vi "Weather Parse Test.vi"() -> ()   [LabVIEW 2020, in "CDM-Config.lvlib"] (continued)
                      \"CMAS\"\n                    ],\n                    \"VTEC\": [\n                        \"/O.CON.KDLH.SC.Y.0132.000000T0000Z-251204T1800Z/\"\n                    ],\n                    \"eventEndingTime\": [\n                        \"2025-12-04T12:00:00-06:00\"\n                    ],\n                    \"expiredReferences\": [\n                        \"w-nws.webmaster@noaa.gov,urn:oid:2.49.0.1.840.0.04f9cf691f6928c5262dfbb988fe18619f2f30e0.003.1,2025-12-02T21:23:00-06:00 w-nws.webmaster@noaa.gov,urn:oid:2.49.0.1.840.0.d19370faedd72659268a7c7b3bafbf3617bad502.003.1,2025-12-02T15:02:00-06:00 w-nws.webmaster@noaa.gov,urn:oid:2.49.0.1.840.0.21fbf4d0662dfb62d7facea472c0c3fe427de6a4.001.1,2025-12-02T09:49:00-06:00\"\n                    ]\n                },\n                \"scope\": \"Public\",\n                \"code\": \"IPAWSv1.0\",\n                \"language\": \"en-US\",\n                \"web\": \"http://www.weather.gov\",\n                \"eventCode\": {\n                    \"SAME\": [\n                        \"NWS\"\n                    ],\n                    \"NationalWeatherService\": [\n                        \"SCY\"\n                    ]\n                }\n            }\n        },\n        {\n            \"id\": \"https://api.weather.gov/alerts/urn:oid:2.49.0.1.840.0.4a9c30a731508078f0f7520ff08e9f1f7a671578.003.2\",\n            \"type\": \"Feature\",\n            \"geometry\": null,\n            \"properties\": {\n                \"@id\": \"https://api.weather.gov/alerts/urn:oid:2.49.0.1.840.0.4a9c30a731508078f0f7520ff08e9f1f7a671578.003.2\",\n                \"@type\": \"wx:Alert\",\n                \"id\": \"urn:oid:2.49.0.1.840.0.4a9c30a731508078f0f7520ff08e9f1f7a671578.003.2\",\n                \"areaDesc\": \"Silver Bay Harbor to Two Harbors MN; Two Harbors to Duluth MN\",\n                \"geocode\": {\n                    \"SAME\": [\n                        \"091143\",\n                        \"091144\"\n                    ],\n                    \"UGC\": [\n                        \"LSZ143\",\n                        \"LSZ144\"\n                    ]\n                },\n                \"affectedZones\": [\n                    \"https://api.weather.gov/zones/forecast/LSZ143\",\n                    \"https://api.weather.gov/zones/forecast/LSZ144\"\n                ],\n                \"references\": [\n                    {\n                        \"@id\": \"https://api.weather.gov/alerts/urn:oid:2.49.0.1.840.0.2b3611bf51a8d91812a27a6d34dc1646d3578776.003.2\",\n                        \"identifier\": \"urn:oid:2.49.0.1.840.0.2b3611bf51a8d91812a27a6d34dc1646d3578776.003.2\",\n                        \"sender\": \"w-nws.webmaster@noaa.gov\",\n                        \"sent\": \"2025-12-03T04:05:00-06:00\"\n                    }\n                ],\n                \"sent\": \"2025-12-03T09:55:00-06:00\",\n                \"effective\": \"2025-12-03T09:55:00-06:00\",\n                \"onset\": \"2025-12-04T12:00:00-06:00\",\n                \"expires\": \"2025-12-03T22:00:00-06:00\",\n                \"ends\": \"2025-12-05T00:00:00-06:00\",\n                \"status\": \"Actual\",\n                \"messageType\": \"Update\",\n                \"category\": \"Met\",\n                \"severity\": \"Moderate\",\n                \"certainty\": \"Possible\",\n                \"urgency\": \"Future\",\n                \"event\": \"Gale Watch\",\n                \"sender\": \"w-nws.webmaster@noaa.gov\",\n                \"senderName\": \"NWS Duluth MN\",\n                \"headline\": \"Gale Watch issued December 3 at 9:55AM CST until December 5 at 12:00AM CST by NWS Duluth MN\",\n                \"description\": \"* WHAT...For the Small Craft Advisory, west winds 10 to 20 kt\\nwith gusts up to 25 kt and waves 1 to 2 ft. For the Gale\\nWatch, southwest winds 15 to 25 kt with gusts up to 35 kt and\\nwaves 3 to 6 ft possible.\\n\\n* WHERE...Silver Bay Harbor to Two Harbors MN and Two Harbors to\\nDuluth MN.\\n\\n* WHEN...For the Small Craft Advisory, until noon CST Thursday.\\nFor the Gale Watch, from Thursday afternoon through Thursday\\nevening.\\n\\n* IMPACTS...Strong winds can cause hazardous waves which could\\ncapsize or damage vessels and reduce visibility.\\n\\n* ADDITIONAL DETAILS...Wind gusts may drop below 20 knots for a\\ntime early this morning and again Thursday morning.\",\n                \"instruction\": \"Mariners should consider altering plans to avoid possible\\nhazardous conditions.  Remain in port, seek safe harbor, alter\\ncourse, and/or secure the vessel for severe wind and waves.\",\n                \"response\": \"Prepare\",\n                \"parameters\": {\n                    \"AWIPSidentifier\": [\n                        \"MWWDLH\"\n                    ],\n                    \"WMOidentifier\": [\n                        \"WHUS73 KDLH 031555\"\n                    ],\n                    \"NWSheadline\": [\n                        \"SMALL CRAFT ADVISORY REMAINS IN EFFECT UNTIL NOON CST THURSDAY... ...GALE WATCH REMAINS IN EFFECT FROM THURSDAY AFTERNOON THROUGH THURSDAY EVENING\"\n                    ],\n                    \"BLOCKCHANNEL\": [\n                        \"EAS\",\n                        \"NWEM\",\n                        \"CMAS\"\n                    ],\n                    \"VTEC\": [\n                        \"/O.CON.KDLH.GL.A.0018.251204T1800Z-251205T0600Z/\"\n                    ],\n                    \"eventEndingTime\": [\n                        \"2025-12-05T00:00:00-06:00\"\n                    ],\n                    \"expiredReferences\": [\n                        \"w-nws.webmaster@noaa.gov,urn:oid:2.49.0.1.840.0.04f9cf691f6928c5262dfbb988fe18619f2f30e0.003.2,2025-12-02T21:23:00-06:00\"\n                    ]\n                },\n                \"scope\": \"Public\",\n                \"code\": \"IPAWSv1.0\",\n                \"language\": \"en-US\",\n                \"web\": \"http://www.weather.gov\",\n                \"eventCode\": {\n                    \"SAME\": [\n                        \"NWS\"\n                    ],\n                    \"NationalWeatherService\": [\n                        \"GLA\"\n                    ]\n                }\n            }\n        },\n        {\n            \"id\": \"https://api.weather.gov/alerts/urn:oid:2.49.0.1.840.0.4a9c30a731508078f0f7520ff08e9f1f7a671578.002.2\",\n            \"type\": \"Feature\",\n            \"geometry\": null,\n            \"properties\": {\n                \"@id\": \"https://api.weather.gov/alerts/urn:oid:2.49.0.1.840.0.4a9c30a731508078f0f7520ff08e9f1f7a671578.002.2\",\n                \"@type\": \"wx:Alert\",\n                \"id\": \"urn:oid:2.49.0.1.840.0.4a9c30a731508078f0f7520ff08e9f1f7a671578.002.2\",\n                \"areaDesc\": \"Grand Portage to Grand Marais MN; Grand Marais to Taconite Harbor MN; Taconite Harbor to Silver Bay Harbor MN\",\n                \"geocode\": {\n                    \"SAME\": [\n                        \"091140\",\n                        \"091141\",\n                        \"091142\"\n                    ],\n                    \"UGC\": [\n                        \"LSZ140\",\n                        \"LSZ141\",\n                        \"LSZ142\"\n                    ]\n                },\n                \"affectedZones\": [\n                    \"https://api.weather.gov/zones/forecast/LSZ140\",\n                    \"https://api.weather.gov/zones/forecast/LSZ141\",\n                    \"https://api.weather.gov/zones/forecast/LSZ142\"\n                ],\n                \"references\": [\n                    {\n                        \"@id\": \"https://api.weather.gov/alerts/urn:oid:2.49.0.1.840.0.2b3611bf51a8d91812a27a6d34dc1646d3578776.002.2\",\n                        \"identifier\": \"urn:oid:2.49.0.1.840.0.2b3611bf51a8d91812a27a6d34dc1646d3578776.002.2\",\n                        \"sender\": \"w-nws.webmaster@noaa.gov\",\n                        \"sent\": \"2025-12-03T04:05:00-06:00\"\n                    }\n                ],\n                \"sent\": \"2025-12-03T09:55:00-06:00\",\n                \"effective\": \"2025-12-03T09:55:00-06:00\",\n                \"onset\": \"2025-12-04T12:00:00-06:00\",\n                \"expires\": \"2025-12-03T22:00:00-06:00\",\n                \"ends\": \"2025-12-05T00:00:00-06:00\",\n                \"status\": \"Actual\",\n                \"messageType\": \"Update\",\n                \"category\": \"Met\",\n                \"severity\": \"Moderate\",\n                \"certainty\": \"Possible\",\n                \"urgency\": \"Future\",\n                \"event\": \"Gale Watch\",\n                \"sender\": \"w-nws.webmaster@noaa.gov\",\n                \"senderName\": \"NWS Duluth MN\",\n                \"headline\": \"Gale Watch issued December 3 at 9:55AM CST until December 5 at 12:00AM CST by NWS Duluth MN\",\n                \"description\": \"* WHAT...For the Small Craft Advisory, northwest winds 10 to 20\\nkt with gusts up to 30 kt and waves 1 to 2 ft. For the Gale\\nWatch, southwest winds 15 to 25 kt with gusts up to 35 kt and\\nwaves 6 to 9 ft possible.\\n\\n* WHERE...Grand Portage to Grand Marais MN, Grand Marais to\\nTaconite Harbor MN and Taconite Harbor to Silver Bay Harbor MN.\\n\\n* WHEN...For the Small Craft Advisory, until noon CST Thursday.\\nFor the Gale Watch, from Thursday afternoon through Thursday\\nevening.\\n\\n* IMPACTS...Strong winds can cause hazardous waves which could\\ncapsize or damage vessels and reduce visibility.\\n\\n* ADDITIONAL DETAILS...Wind gusts may drop below 20 knots for a\\ntime early this morning and again Thursday morning.\",\n                \"instruction\": \"Mariners should consider altering plans to avoid possible\\nhazardous conditions.  Remain in port, seek safe harbor, alter\\ncourse, and/or secure the vessel for severe wind and waves.\",\n                \"response\": \"Prepare\",\n                \"parameters\": {\n                    \"AWIPSidentifier\": [\n                        \"MWWDLH\"\n                    ],\n                    \"WMOidentifier\": [\n                        \"WHUS73 KDLH 031555\"\n                    ],\n                    \"NWSheadline\": [\n                        \"SMALL CRAFT ADVISORY REMAINS IN EFFECT UNTIL NOON CST THURSDAY... ...GALE WATCH REMAINS IN EFFECT FROM THURSDAY AFTERNOON THROUGH THURSDAY EVENING\"\n                    ],\n                    \"BLOCKCHANNEL\": [\n                        \"EAS\",\n                        \"NWEM\",\n                        \"CMAS\"\n                    ],\n                    \"VTEC\": [\n                        \"/O.CON.KDLH.GL.A.0018.251204T1800Z-251205T0600Z/\"\n                    ],\n                    \"eventEndingTime\": [\n                        \"2025-12-05T00:00:00-06:00\"\n                    ],\n                    \"expiredReferences\": [\n                        \"w-nws.webmaster@noaa.gov,urn:oid:2.49.0.1.840.0.04f9cf691f6928c5262dfbb988fe18619f2f30e0.002.2,2025-12-02T21:23:00-06:00\"\n                    ]\n                },\n                \"scope\": \"Public\",\n                \"code\": \"IPAWSv1.0\",\n                \"language\": \"en-US\",\n                \"web\": \"http://www.weather.gov\",\n                \"eventCode\": {\n                    \"SAME\": [\n                        \"NWS\"\n                    ],\n                    \"NationalWeatherService\": [\n                        \"GLA\"\n                    ]\n                }\n            }\n        },\n        {\n            \"id\": \"https://api.weather.gov/alerts/urn:oid:2.49.0.1.840.0.4a9c30a731508078f0f7520ff08e9f1f7a671578.004.1\",\n            \"type\": \"Feature\",\n            \"geometry\": null,\n            \"properties\": {\n                \"@id\": \"https://api.weather.gov/alerts/urn:oid:2.49.0.1.840.0.4a9c30a731508078f0f7520ff08e9f1f7a671578.004.1\",\n                \"@type\": \"wx:Alert\",\n                \"id\": \"urn:oid:2.49.0.1.840.0.4a9c30a731508078f0f7520ff08e9f1f7a671578.004.1\",\n                \"areaDesc\": \"Chequamegon Bay-Bayfield to Oak Point WI; Duluth MN to Port Wing WI; Port Wing to Sand Island WI; Sand Island to Bayfield WI; Oak Point to Saxon Harbor WI\",\n                \"geocode\": {\n                    \"SAME\": [\n                        \"091121\",\n                        \"091145\",\n                        \"091146\",\n                        \"091147\",\n                        \"091148\"\n                    ],\n                    \"UGC\": [\n                        \"LSZ121\",\n                        \"LSZ145\",\n                        \"LSZ146\",\n                        \"LSZ147\",\n                        \"LSZ148\"\n                    ]\n                },\n                \"affectedZones\": [\n                    \"https://api.weather.gov/zones/forecast/LSZ121\",\n                    \"https://api.weather.gov/zones/forecast/LSZ145\",\n                    \"https://api.weather.gov/zones/forecast/LSZ146\",\n                    \"https://api.weather.gov/zones/forecast/LSZ147\",\n                    \"https://api.weather.gov/zones/forecast/LSZ148\"\n                ],\n                \"references\": [\n                    {\n                        \"@id\": \"https://api.weather.gov/alerts/urn:oid:2.49.0.1.840.0.2b3611bf51a8d91812a27a6d34dc1646d3578776.004.1\",\n                        \"identifier\": \"urn:oid:2.49.0.1.840.0.2b3611bf51a8d91812a27a6d34dc1646d3578776.004.1\",\n                        \"sender\": \"w-nws.webmaster@noaa.gov\",\n                        \"sent\": \"2025-12-03T04:05:00-06:00\"\n                    }\n                ],\n                \"sent\": \"2025-12-03T09:55:00-06:00\",\n                \"effective\": \"2025-12-03T09:55:00-06:00\",\n                \"onset\": \"2025-12-03T09:55:00-06:00\",\n                \"expires\": \"2025-12-03T22:00:00-06:00\",\n                \"ends\": \"2025-12-05T10:00:00-06:00\",\n                \"status\": \"Actual\",\n                \"messageType\": \"Update\",\n                \"category\": \"Met\",\n                \"severity\": \"Minor\",\n                \"certainty\": \"Likely\",\n                \"urgency\": \"Expected\",\n                \"event\": \"Small Craft Advisory\",\n                \"sender\": \"w-nws.webmaster@noaa.gov\",\n                \"senderName\": \"NWS Duluth MN\",\n                \"headline\": \"Small Craft Advisory issued December 3 at 9:55AM CST until December 5 at 10:00AM CST by NWS Duluth MN\",\n                \"description\": \"* WHAT...West winds 15 to 25 kt with gusts up to 35 kt and waves\\n2 to 5 ft.\\n\\n* WHERE...Chequamegon Bay-Bayfield to Oak Point WI, Duluth MN to\\nPort Wing WI, Port Wing to Sand Island WI, Sand Island to\\nBayfield WI and Oak Point to Saxon Harbor WI.\\n\\n* WHEN...Until 10 AM CST Friday.\\n\\n* IMPACTS...Conditions will be hazardous to small craft.\\n\\n* ADDITIONAL DETAILS...Wind gusts may drop below 20 knots for a\\ntime early this morning and again Thursday morning.\",\n                \"instruction\": \"Anyone operating a smaller vessel should avoid navigating in\\nhazardous conditions.\",\n                \"response\": \"Avoid\",\n                \"parameters\": {\n                    \"AWIPSidentifier\": [\n                        \"MWWDLH\"\n                    ],\n                    \"WMOidentifier\": [\n                        \"WHUS73 KDLH 031555\"\n                    ],\n                    \"NWSheadline\": [\n                        \"SMALL CRAFT ADVISORY REMAINS IN EFFECT UNTIL 10 AM CST FRIDAY\"\n                    ],\n                    \"BLOCKCHANNEL\": [\n                        \"EAS\",\n                        \"NWEM\",\n                        \"CMAS\"\n                    ],\n                    \"VTEC\": [\n                        \"/O.CON.KDLH.SC.Y.0132.000000T0000Z-251205T1600Z/\"\n                    ],\n                    \"eventEndingTime\": [\n                        \"2025-12-05T10:00:00-06:00\"\n                    ],\n                    \"expiredReferences\": [\n                        \"w-nws.webmaster@noaa.gov,urn:oid:2.49.0.1.840.0.04f9cf691f6928c5262dfbb988fe18619f2f30e0.004.1,2025-12-02T21:23:00-06:00 w-nws.webmaster@noaa.gov,urn:oid:2.49.0.1.840.0.d19370faedd72659268a7c7b3bafbf3617bad502.003.1,2025-12-02T15:02:00-06:00 w-nws.webmaster@noaa.gov,urn:oid:2.49.0.1.840.0.21fbf4d0662dfb62d7facea472c0c3fe427de6a4.001.1,2025-12-02T09:49:00-06:00\"\n                    ]\n                },\n                \"scope\": \"Public\",\n                \"code\": \"IPAWSv1.0\",\n                \"language\": \"en-US\",\n                \"web\": \"http://www.weather.gov\",\n                \"eventCode\": {\n                    \"SAME\": [\n                        \"NWS\"\n                    ],\n                    \"NationalWeatherService\": [\n                        \"SCY\"\n                    ]\n                }\n            }\n        },\n        {\n            \"id\": \"https://api.weather.gov/alerts/urn:oid:2.49.0.1.840.0.cb3741455a35586feac70bfcfc92a33545eb4f89.001.1\",\n            \"type\": \"Feature\",\n            \"geometry\": null,\n            \"properties\": {\n                \"@id\": \"https://api.weather.gov/alerts/urn:oid:2.49.0.1.840.0.cb3741455a35586feac70bfcfc92a33545eb4f89.001.1\",\n                \"@type\": \"wx:Alert\",\n                \"id\": \"urn:oid:2.49.0.1.840.0.cb3741455a35586feac70bfcfc92a33545eb4f89.001.1\",\n                \"areaDesc\": \"Southern Blue Mountains of Oregon; John Day Basin; Ochoco-John Day Highlands; North Central Oregon\",\n                \"geocode\": {\n                    \"SAME\": [\n                        \"041021\",\n                        \"041023\",\n                        \"041049\",\n                        \"041059\",\n                        \"041061\",\n                        \"041069\",\n                        \"041031\",\n                        \"041065\",\n                        \"041013\",\n                        \"041017\",\n                        \"041055\"\n                    ],\n                    \"UGC\": [\n                        \"ORZ503\",\n                        \"ORZ505\",\n                        \"ORZ506\",\n                        \"ORZ510\"\n                    ]\n                },\n                \"affectedZones\": [\n                    \"https://api.weather.gov/zones/forecast/ORZ503\",\n                    \"https://api.weather.gov/zones/forecast/ORZ505\",\n                    \"https://api.weather.gov/zones/forecast/ORZ506\",\n                    \"https://api.weather.gov/zones/forecast/ORZ510\"\n                ],\n                \"references\": [],\n                \"sent\": \"2025-12-03T07:47:00-08:00\",\n                \"effective\": \"2025-12-03T07:47:00-08:00\",\n                \"onset\": \"2025-12-03T07:47:00-08:00\",\n                \"expires\": \"2025-12-03T13:00:00-08:00\",\n                \"ends\": null,\n                \"status\": \"Actual\",\n                \"messageType\": \"Alert\",\n                \"category\": \"Met\",\n                \"severity\": \"Moderate\",\n                \"certainty\": \"Observed\",\n                \"urgency\": \"Expected\",\n                \"event\": \"Special Weather Statement\",\n                \"sender\": \"w-nws.webmaster@noaa.gov\",\n                \"senderName\": \"NWS Pendleton OR\",\n                \"headline\": \"Special Weather Statement issued December 3 at 7:47AM PST by NWS Pendleton OR\",\n                \"description\": \"Patchy dense freezing fog has been observed on local traffic and\\nwildfire cameras, with visibilities estimated to be less than a\\nmile and temperatures below freezing in some of these areas. Area\\nhighways that are being impacted include US Highways 395, 97,\\n197, 26, and 20, as well as Oregon Highways 218, 216, 208, 207,\\n206, 74, and 19. Reduced visibilities and ice accretion on\\nroadways may impact travel. The freezing fog will lift by this\\nafternoon.\",\n                \"instruction\": null,\n                \"response\": \"Execute\",\n                \"parameters\": {\n                    \"AWIPSidentifier\": [\n                        \"SPSPDT\"\n                    ],\n                    \"WMOidentifier\": [\n                        \"WWUS86 KPDT 031547\"\n                    ],\n                    \"BLOCKCHANNEL\": [\n                        \"EAS\",\n                        \"NWEM\",\n                        \"CMAS\"\n                    ],\n                    \"EAS-ORG\": [\n                        \"WXR\"\n                    ]\n                },\n                \"scope\": \"Public\",\n                \"code\": \"IPAWSv1.0\",\n                \"language\": \"en-US\",\n                \"web\": \"http://www.weather.gov\",\n                \"eventCode\": {\n                    \"SAME\": [\n                        \"SPS\"\n                    ],\n                    \"NationalWeatherService\": [\n                        \"SPS\"\n                    ]\n                }\n            }\n        },\n        {\n            \"id\": \"https://api.weather.gov/alerts/urn:oid:2.49.0.1.840.0.d69e0fdad84e1f558091761919060d14ba7d6a4a.001.1\",\n            \"type\": \"Feature\",\n            \"geometry\": null,\n            \"properties\": {\n                \"@id\": \"https://api.weather.gov/alerts/urn:oid:2.49.0.1.840.0.d69e0fdad84e1f558091761919060d14ba7d6a4a.001.1\",\n                \"@type\": \"wx:Alert\",\n                \"id\": \"urn:oid:2.49.0.1.840.0.d69e0fdad84e1f558091761919060d14ba7d6a4a.001.1\",\n                \"areaDesc\": \"Grand Traverse Bay south of a line Grand Traverse Light to Norwood MI; Seul Choix Point to 5NM West of Mackinac Bridge; Norwood MI to 5NM West of Mackinac Bridge including Little Traverse Bay; Sleeping Bear Point to Grand Traverse Light MI; Point Betsie to Sleeping Bear Point MI; Manistee to Point Betsie MI\",\n                \"geocode\": {\n                    \"SAME\": [\n                        \"092323\",\n                        \"092341\",\n                        \"092342\",\n                        \"092344\",\n                        \"092345\",\n                        \"092346\"\n                    ],\n                    \"UGC\": [\n                        \"LMZ323\",\n                        \"LMZ341\",\n                        \"LMZ342\",\n                        \"LMZ344\",\n                        \"LMZ345\",\n                        \"LMZ346\"\n                    ]\n                },\n                \"affectedZones\": [\n                    \"https://api.weather.gov/zones/forecast/LMZ323\",\n                    \"https://api.weather.gov/zones/forecast/LMZ341\",\n                    \"https://api.weather.gov/zones/forecast/LMZ342\",\n                    \"https://api.weather.gov/zones/forecast/LMZ344\",\n                    \"https://api.weather.gov/zones/forecast/LMZ345\",\n                    \"https://api.weather.gov/zones/forecast/LMZ346\"\n                ],\n                \"references\": [\n                    {\n                        \"@id\": \"https://api.weather.gov/alerts/urn:oid:2.49.0.1.840.0.d4f341bf09774259e03e3637f08a5e0369a8be29.001.1\",\n                        \"identifier\": \"urn:oid:2.49.0.1.840.0.d4f341bf09774259e03e3637f08a5e0369a8be29.001.1\",\n                        \"sender\": \"w-nws.webmaster@noaa.gov\",\n                        \"sent\": \"2025-12-03T02:58:00-05:00\"\n                    }\n                ],\n                \"sent\": \"2025-12-03T10:45:00-05:00\",\n                \"effective\": \"2025-12-03T10:45:00-05:00\",\n                \"onset\": \"2025-12-03T10:45:00-05:00\",\n                \"expires\": \"2025-12-03T19:45:00-05:00\",\n                \"ends\": \"2025-12-04T13:00:00-05:00\",\n                \"status\": \"Actual\",\n                \"messageType\": \"Update\",\n                \"category\": \"Met\",\n                \"severity\": \"Minor\",\n                \"certainty\": \"Likely\",\n                \"urgency\": \"Expected\",\n                \"event\": \"Small Craft Advisory\",\n                \"sender\": \"w-nws.webmaster@noaa.gov\",\n                \"senderName\": \"NWS Gaylord MI\",\n                \"headline\": \"Small Craft Advisory issued December 3 at 10:45AM EST until December 4 at 1:00PM EST by NWS Gaylord MI\",\n                \"description\": \"* WHAT...For the Small Craft Advisory, Highest gusts up to 30\\nkts from the northwest and highest waves around 8 feet. For\\nthe Gale Watch, Highest gusts up to 45 kts from the southwest\\nand highest waves around 13 feet possible.\\n\\n* WHERE...Portions of Lake Michigan.\\n\\n* WHEN...For the Small Craft Advisory, until 1 PM EST Thursday.\\nFor the Gale Watch, from Thursday evening through Friday\\nmorning.\\n\\n* IMPACTS...Strong winds can cause hazardous highest waves which\\ncould capsize or damage vessels and reduce visibility.\",\n                \"instruction\": \"Mariners should consider altering plans to avoid possible\\nhazardous conditions.  Remain in port, seek safe harbor, alter\\ncourse, and/or secure the vessel for severe wind and highest\\nwaves.\",\n                \"response\": \"Avoid\",\n                \"parameters\": {\n                    \"AWIPSidentifier\": [\n                        \"MWWAPX\"\n                    ],\n                    \"WMOidentifier\": [\n                        \"WHUS73 KAPX 031545\"\n                    ],\n                    \"NWSheadline\": [\n                        \"SMALL CRAFT ADVISORY REMAINS IN EFFECT UNTIL 1 PM EST THURSDAY... ...GALE WATCH REMAINS IN EFFECT FROM THURSDAY EVENING THROUGH FRIDAY MORNING\"\n                    ],\n                    \"BLOCKCHANNEL\": [\n                        \"EAS\",\n                        \"NWEM\",\n                        \"CMAS\"\n                    ],\n                    \"VTEC\": [\n                        \"/O.CON.KAPX.SC.Y.0118.000000T0000Z-251204T1800Z/\"\n                    ],\n                    \"eventEndingTime\": [\n                        \"2025-12-04T13:00:00-05:00\"\n                    ],\n                    \"expiredReferences\": [\n                        \"w-nws.webmaster@noaa.gov,urn:oid:2.49.0.1.840.0.db358447f299fb9ab627f5ec5bd8edba51730923.002.1,2025-12-02T23:15:00-05:00 w-nws.webmaster@noaa.gov,urn:oid:2.49.0.1.840.0.dbbd5f9aa1adb1588c67ea3394dc6c72c6a93051.001.1,2025-12-02T14:38:00-05:00 w-nws.webmaster@noaa.gov,urn:oid:2.49.0.1.840.0.bcebcfef404dc927a35a81355eb23e28922a6e4b.001.1,2025-12-02T10:30:00-05:00 w-nws.webmaster@noaa.gov,urn:oid:2.49.0.1.840.0.0625dac845521af5ccf69b7232976b528a83340a.001.1,2025-12-02T02:46:00-05:00\"\n                    ]\n                },\n                \"scope\": \"Public\",\n                \"code\": \"IPAWSv1.0\",\n                \"language\": \"en-US\",\n                \"web\": \"http://www.weather.gov\",\n                \"eventCode\": {\n                    \"SAME\": [\n                        \"NWS\"\n                    ],\n                    \"NationalWeatherService\": [\n                        \"SCY\"\n                    ]\n                }\n            }\n        },\n        {\n            \"id\": \"https://api.weather.gov/alerts/urn:oid:2.49.0.1.840.0.d69e0fdad84e1f558091761919060d14ba7d6a4a.003.1\",\n            \"type\": \"Feature\",\n            \"geometry\": null,\n            \"properties\": {\n                \"@id\": \"https://api.weather.gov/alerts/urn:oid:2.49.0.1.840.0.d69e0fdad84e1f558091761919060d14ba7d6a4a.003.1\",\n                \"@type\": \"wx:Alert\",\n                \"id\": \"urn:oid:2.49.0.1.840.0.d69e0fdad84e1f558091761919060d14ba7d6a4a.003.1\",\n                \"areaDesc\": \"Straits of Mackinac within 5 nm of Mackinac Bridge including Mackinac Island; St Ignace to False Detour Channel; 5NM East of Mackinac Bridge to Presque Isle Light MI including Bois Blanc Island; Presque Isle Light to Sturgeon Pt MI Including Thunder Bay National Marine Sanctuary; Sturgeon Pt to Alabaster MI\",\n                \"geocode\": {\n                    \"SAME\": [\n                        \"093345\",\n                        \"093346\",\n                        \"093347\",\n                        \"093348\",\n                        \"093349\"\n                    ],\n                    \"UGC\": [\n                        \"LHZ345\",\n                        \"LHZ346\",\n                        \"LHZ347\",\n                        \"LHZ348\",\n                        \"LHZ349\"\n                    ]\n                },\n                \"affectedZones\": [\n                    \"https://api.weather.gov/zones/forecast/LHZ345\",\n                    \"https://api.weather.gov/zones/forecast/LHZ346\",\n                    \"https://api.weather.gov/zones/forecast/LHZ347\",\n                    \"https://api.weather.gov/zones/forecast/LHZ348\",\n                    \"https://api.weather.gov/zones/forecast/LHZ349\"\n                ],\n                \"references\": [\n                    {\n                        \"@id\": \"https://api.weather.gov/alerts/urn:oid:2.49.0.1.840.0.d4f341bf09774259e03e3637f08a5e0369a8be29.003.1\",\n                        \"identifier\": \"urn:oid:2.49.0.1.840.0.d4f341bf09774259e03e3637f08a5e0369a8be29.003.1\",\n                        \"sender\": \"w-nws.webmaster@noaa.gov\",\n                        \"sent\": \"2025-12-03T02:58:00-05:00\"\n                    }\n                ],\n                \"sent\": \"2025-12-03T10:45:00-05:00\",\n                \"effective\": \"2025-12-03T10:45:00-05:00\",\n                \"onset\": \"2025-12-03T10:45:00-05:00\",\n                \"expires\": \"2025-12-03T19:45:00-05:00\",\n                \"ends\": \"2025-12-04T13:00:00-05:00\",\n                \"status\": \"Actual\",\n                \"messageType\": \"Update\",\n                \"category\": \"Met\",\n                \"severity\": \"Minor\",\n                \"certainty\": \"Likely\",\n                \"urgency\": \"Expected\",\n                \"event\": \"Small Craft Advisory\",\n                \"sender\": \"w-nws.webmaster@noaa.gov\",\n                \"senderName\": \"NWS Gaylord MI\",\n                \"headline\": \"Small Craft Advisory issued December 3 at 10:45AM EST until December 4 at 1:00PM EST by NWS Gaylord MI\",\n                \"description\": \"* WHAT...Highest gusts up to 30 kts from the northwest and\\nhighest waves around 9 feet.\\n\\n* WHERE...Straits of Mackinac within 5 nm of Mackinac Bridge\\nincluding Mackinac Island, St Ignace to False Detour Channel,\\n5NM East of Mackinac Bridge to Presque Isle Light MI including\\nBois Blanc Island, Presque Isle Light to Sturgeon Pt MI\\nIncluding Thunder Bay National Marine Sanctuary and Sturgeon\\nPt to Alabaster MI.\\n\\n* WHEN...Until 1 PM EST Thursday.\\n\\n* IMPACTS...Conditions will be hazardous to small craft.\",\n                \"instruction\": \"Inexperienced mariners, especially those operating smaller\\nvessels, should avoid navigating in hazardous conditions.\",\n                \"response\": \"Avoid\",\n                \"parameters\": {\n                    \"AWIPSidentifier\": [\n                        \"MWWAPX\"\n                    ],\n                    \"WMOidentifier\": [\n                        \"WHUS73 KAPX 031545\"\n                    ],\n                    \"NWSheadline\": [\n                        \"SMALL CRAFT ADVISORY REMAINS IN EFFECT UNTIL 1 PM EST THURSDAY\"\n                    ],\n                    \"BLOCKCHANNEL\": [\n                        \"EAS\",\n                        \"NWEM\",\n                        \"CMAS\"\n                    ],\n                    \"VTEC\": [\n                        \"/O.CON.KAPX.SC.Y.0118.000000T0000Z-251204T1800Z/\"\n                    ],\n                    \"eventEndingTime\": [\n                        \"2025-12-04T13:00:00-05:00\"\n                    ],\n                    \"expiredReferences\": [\n                        \"w-nws.webmaster@noaa.gov,urn:oid:2.49.0.1.840.0.db358447f299fb9ab627f5ec5bd8edba51730923.004.1,2025-12-02T23:15:00-05:00 w-nws.webmaster@noaa.gov,urn:oid:2.49.0.1.840.0.dbbd5f9aa1adb1588c67ea3394dc6c72c6a93051.003.1,2025-12-02T14:38:00-05:00 w-nws.webmaster@noaa.gov,urn:oid:2.49.0.1.840.0.bcebcfef404dc927a35a81355eb23e28922a6e4b.003.1,2025-12-02T10:30:00-05:00 w-nws.webmaster@noaa.gov,urn:oid:2.49.0.1.840.0.0625dac845521af5ccf69b7232976b528a83340a.003.1,2025-12-02T02:46:00-05:00\"\n                    ]\n                },\n                \"scope\": \"Public\",\n                \"code\": \"IPAWSv1.0\",\n                \"language\": \"en-US\",\n                \"web\": \"http://www.weather.gov\",\n                \"eventCode\": {\n                    \"SAME\": [\n                        \"NWS\"\n                    ],\n                    \"NationalWeatherService\": [\n                        \"SCY\"\n                    ]\n                }\n            }\n        },\n        {\n            \"id\": \"https://api.weather.gov/alerts/urn:oid:2.49.0.1.840.0.d69e0fdad84e1f558091761919060d14ba7d6a4a.002.1\",\n            \"type\": \"Feature\",\n            \"geometry\": null,\n            \"properties\": {\n                \"@id\": \"https://api.weather.gov/alerts/urn:oid:2.49.0.1.840.0.d69e0fdad84e1f558091761919060d14ba7d6a4a.002.1\",\n                \"@type\": \"wx:Alert\",\n                \"id\": \"urn:oid:2.49.0.1.840.0.d69e0fdad84e1f558091761919060d14ba7d6a4a.002.1\",\n                \"areaDesc\": \"Whitefish Bay (U.S. Portion)/Whitefish Point to Point Iroquois MI; St. Marys River Point Iroquois to E. Potagannissing Bay\",\n                \"geocode\": {\n                    \"SAME\": [\n                        \"091321\",\n                        \"091322\"\n                    ],\n                    \"UGC\": [\n                        \"LSZ321\",\n                        \"LSZ322\"\n                    ]\n                },\n                \"affectedZones\": [\n                    \"https://api.weather.gov/zones/forecast/LSZ321\",\n                    \"https://api.weather.gov/zones/forecast/LSZ322\"\n                ],\n                \"references\": [\n                    {\n                        \"@id\": \"https://api.weather.gov/alerts/urn:oid:2.49.0.1.840.0.d4f341bf09774259e03e3637f08a5e0369a8be29.002.1\",\n                        \"identifier\": \"urn:oid:2.49.0.1.840.0.d4f341bf09774259e03e3637f08a5e0369a8be29.002.1\",\n                        \"sender\": \"w-nws.webmaster@noaa.gov\",\n                        \"sent\": \"2025-12-03T02:58:00-05:00\"\n                    }\n                ],\n                \"sent\": \"2025-12-03T10:45:00-05:00\",\n                \"effective\": \"2025-12-03T10:45:00-05:00\",\n                \"onset\": \"2025-12-03T10:45:00-05:00\",\n                \"expires\": \"2025-12-03T19:45:00-05:00\",\n                \"ends\": \"2025-12-04T13:00:00-05:00\",\n                \"status\": \"Actual\",\n                \"messageType\": \"Update\",\n                \"category\": \"Met\",\n                \"severity\": \"Minor\",\n                \"certainty\": \"Likely\",\n                \"urgency\": \"Expected\",\n                \"event\": \"Small Craft Advisory\",\n                \"sender\": \"w-nws.webmaster@noaa.gov\",\n                \"senderName\": \"NWS Gaylord MI\",\n                \"headline\": \"Small Craft Advisory issued December 3 at 10:45AM EST until December 4 at 1:00PM EST by NWS Gaylord MI\",\n                \"description\": \"* WHAT...Highest gusts up to 30 kts from the northwest and\\nhighest waves around 10 feet.\\n\\n* WHERE...Whitefish Bay (U. S. Portion)/Whitefish Point to Point\\nIroquois MI and St. Marys River Point Iroquois to E.\\nPotagannissing Bay.\\n\\n* WHEN...Until 1 PM EST Thursday.\\n\\n* IMPACTS...Conditions will be hazardous to small craft.\",\n                \"instruction\": \"Inexperienced mariners, especially those operating smaller\\nvessels, should avoid navigating in hazardous conditions.\",\n                \"response\": \"Avoid\",\n                \"parameters\": {\n                    \"AWIPSidentifier\": [\n                        \"MWWAPX\"\n                    ],\n                    \"WMOidentifier\": [\n                        \"WHUS73 KAPX 031545\"\n                    ],\n                    \"NWSheadline\": [\n                        \"SMALL CRAFT ADVISORY REMAINS IN EFFECT UNTIL 1 PM EST THURSDAY\"\n                    ],\n                    \"BLOCKCHANNEL\": [\n                        \"EAS\",\n                        \"NWEM\",\n                        \"CMAS\"\n                    ],\n                    \"VTEC\": [\n                        \"/O.CON.KAPX.SC.Y.0118.000000T0000Z-251204T1800Z/\"\n                    ],\n                    \"eventEndingTime\": [\n                        \"2025-12-04T13:00:00-05:00\"\n                    ],\n                    \"expiredReferences\": [\n                        \"w-nws.webmaster@noaa.gov,urn:oid:2.49.0.1.840.0.db358447f299fb9ab627f5ec5bd8edba51730923.003.1,2025-12-02T23:15:00-05:00 w-nws.webmaster@noaa.gov,urn:oid:2.49.0.1.840.0.db358447f299fb9ab627f5ec5bd8edba51730923.001.1,2025-12-02T23:15:00-05:00 w-nws.webmaster@noaa.gov,urn:oid:2.49.0.1.840.0.dbbd5f9aa1adb1588c67ea3394dc6c72c6a93051.002.1,2025-12-02T14:38:00-05:00 w-nws.webmaster@noaa.gov,urn:oid:2.49.0.1.840.0.bcebcfef404dc927a35a81355eb23e28922a6e4b.002.1,2025-12-02T10:30:00-05:00 w-nws.webmaster@noaa.gov,urn:oid:2.49.0.1.840.0.0625dac845521af5ccf69b7232976b528a83340a.002.1,2025-12-02T02:46:00-05:00\"\n                    ]\n                },\n                \"scope\": \"Public\",\n                \"code\": \"IPAWSv1.0\",\n                \"language\": \"en-US\",\n                \"web\": \"http://www.weather.gov\",\n                \"eventCode\": {\n                    \"SAME\": [\n                        \"NWS\"\n                    ],\n                    \"NationalWeatherService\": [\n                        \"SCY\"\n                    ]\n                }\n            }\n        },\n        {\n            \"id\": \"https://api.weather.gov/alerts/urn:oid:2.49.0.1.840.0.d69e0fdad84e1f558091761919060d14ba7d6a4a.001.2\",\n            \"type\": \"Feature\",\n            \"geometry\": null,\n            \"properties\": {\n                \"@id\": \"https://api.weather.gov/alerts/urn:oid:2.49.0.1.840.0.d69e0fdad84e1f558091761919060d14ba7d6a4a.001.2\",\n                \"@type\": \"wx:Alert\",\n                \"id\": \"urn:oid:2.49.0.1.840.0.d69e0fdad84e1f558091761919060d14ba7d6a4a.001.2\",\n                \"areaDesc\": \"Grand Traverse Bay south of a line Grand Traverse Light to Norwood MI; Seul Choix Point to 5NM West of Mackinac Bridge; Norwood MI to 5NM West of Mackinac Bridge including Little Traverse Bay; Sleeping Bear Point to Grand Traverse Light MI; Point Betsie to Sleeping Bear Point MI; Manistee to Point Betsie MI\",\n                \"geocode\": {\n                    \"SAME\": [\n                        \"092323\",\n                        \"092341\",\n                        \"092342\",\n                        \"092344\",\n                        \"092345\",\n                        \"092346\"\n                    ],\n                    \"UGC\": [\n                        \"LMZ323\",\n                        \"LMZ341\",\n                        \"LMZ342\",\n                        \"LMZ344\",\n                        \"LMZ345\",\n                        \"LMZ346\"\n                    ]\n                },\n                \"affectedZones\": [\n                    \"https://api.weather.gov/zones/forecast/LMZ323\",\n                    \"https://api.weather.gov/zones/forecast/LMZ341\",\n                    \"https://api.weather.gov/zones/forecast/LMZ342\",\n                    \"https://api.weather.gov/zones/forecast/LMZ344\",\n                    \"https://api.weather.gov/zones/forecast/LMZ345\",\n                    \"https://api.weather.gov/zones/forecast/LMZ346\"\n                ],\n                \"references\": [\n                    {\n                        \"@id\": \"https://api.weather.gov/alerts/urn:oid:2.49.0.1.840.0.d4f341bf09774259e03e3637f08a5e0369a8be29.001.2\",\n                        \"identifier\": \"urn:oid:2.49.0.1.840.0.d4f341bf09774259e03e3637f08a5e0369a8be29.001.2\",\n                        \"sender\": \"w-nws.webmaster@noaa.gov\",\n                        \"sent\": \"2025-12-03T02:58:00-05:00\"\n                    }\n                ],\n                \"sent\": \"2025-12-03T10:45:00-05:00\",\n                \"effective\": \"2025-12-03T10:45:00-05:00\",\n                \"onset\": \"2025-12-04T22:00:00-05:00\",\n                \"expires\": \"2025-12-03T19:45:00-05:00\",\n                \"ends\": \"2025-12-05T07:00:00-05:00\",\n                \"status\": \"Actual\",\n                \"messageType\": \"Update\",\n                \"category\": \"Met\",\n                \"severity\": \"Moderate\",\n                \"certainty\": \"Possible\",\n                \"urgency\": \"Future\",\n                \"event\": \"Gale Watch\",\n                \"sender\": \"w-nws.webmaster@noaa.gov\",\n                \"senderName\": \"NWS Gaylord MI\",\n                \"headline\": \"Gale Watch issued December 3 at 10:45AM EST until December 5 at 7:00AM EST by NWS Gaylord MI\",\n                \"description\": \"* WHAT...For the Small Craft Advisory, Highest gusts up to 30\\nkts from the northwest and highest waves around 8 feet. For\\nthe Gale Watch, Highest gusts up to 45 kts from the southwest\\nand highest waves around 13 feet possible.\\n\\n* WHERE...Portions of Lake Michigan.\\n\\n* WHEN...For the Small Craft Advisory, until 1 PM EST Thursday.\\nFor the Gale Watch, from Thursday evening through Friday\\nmorning.\\n\\n* IMPACTS...Strong winds can cause hazardous highest waves which\\ncould capsize or damage vessels and reduce visibility.\",\n                \"instruction\": \"Mariners should consider altering plans to avoid possible\\nhazardous conditions.  Remain in port, seek safe harbor, alter\\ncourse, and/or secure the vessel for severe wind and highest\\nwaves.\",\n                \"response\": \"Prepare\",\n                \"parameters\": {\n                    \"AWIPSidentifier\": [\n                        \"MWWAPX\"\n                    ],\n                    \"WMOidentifier\": [\n                        \"WHUS73 KAPX 031545\"\n                    ],\n                    \"NWSheadline\": [\n                        \"SMALL CRAFT ADVISORY REMAINS IN EFFECT UNTIL 1 PM EST THURSDAY... ...GALE WATCH REMAINS IN EFFECT FROM THURSDAY EVENING THROUGH FRIDAY MORNING\"\n                    ],\n                    \"BLOCKCHANNEL\": [\n                        \"EAS\",\n                        \"NWEM\",\n                        \"CMAS\"\n                    ],\n                    \"VTEC\": [\n                        \"/O.CON.KAPX.GL.A.0018.251205T0300Z-251205T1200Z/\"\n                    ],\n                    \"eventEndingTime\": [\n                        \"2025-12-05T07:00:00-05:00\"\n                    ]\n                },\n                \"scope\": \"Public\",\n                \"code\": \"IPAWSv1.0\",\n                \"language\": \"en-US\",\n                \"web\": \"http://www.weather.gov\",\n                \"eventCode\": {\n                    \"SAME\": [\n                        \"NWS\"\n                    ],\n                    \"NationalWeatherService\": [\n                        \"GLA\"\n                    ]\n                }\n            }\n        },\n        {\n            \"id\": \"https://api.weather.gov/alerts/urn:oid:2.49.0.1.840.0.537a28e93f92ae0fdb03834109f43a3016f926b7.006.1\",\n            \"type\": \"Feature\",\n            \"geometry\": null,\n            \"properties\": {\n                \"@id\": \"https://api.weather.gov/alerts/urn:oid:2.49.0.1.840.0.537a28e93f92ae0fdb03834109f43a3016f926b7.006.1\",\n                \"@type\": \"wx:Alert\",\n                \"id\": \"urn:oid:2.49.0.1.840.0.537a28e93f92ae0fdb03834109f43a3016f926b7.006.1\",\n                \"areaDesc\": \"Cross Sound\",\n                \"geocode\": {\n                    \"SAME\": [\n                        \"058022\"\n                    ],\n                    \"UGC\": [\n                        \"PKZ022\"\n                    ]\n                },\n                \"affectedZones\": [\n                    \"https://api.weather.gov/zones/forecast/PKZ022\"\n                ],\n                \"references\": [],\n                \"sent\": \"2025-12-03T06:43:00-09:00\",\n                \"effective\": \"2025-12-03T06:43:00-09:00\",\n                \"onset\": \"2025-12-03T06:00:00-09:00\",\n                \"expires\": \"2025-12-03T18:15:00-09:00\",\n                \"ends\": \"2025-12-04T05:00:00-09:00\",\n                \"status\": \"Actual\",\n                \"messageType\": \"Alert\",\n                \"category\": \"Met\",\n                \"severity\": \"Minor\",\n                \"certainty\": \"Likely\",\n                \"urgency\": \"Expected\",\n                \"event\": \"Small Craft Advisory\",\n                \"sender\": \"w-nws.webmaster@noaa.gov\",\n                \"senderName\": \"NWS Juneau AK\",\n                \"headline\": \"Small Craft Advisory issued December 3 at 6:43AM AKST until December 4 at 5:00AM AKST by NWS Juneau AK\",\n                \"description\": \"Southeast Alaska Inside Waters from Dixon Entrance to Skagway\\n\\nWind forecasts reflect the predominant speed and direction\\nexpected. Sea forecasts represent the average of the highest\\none-third of the combined windwave and swell height.\\n\\n.TODAY...E wind 25 kt becoming SW 15 kt in the afternoon. Seas\\n9 ft. Rain.\\n.TONIGHT...SW wind 20 kt. Seas 8 ft. S swell. Rain in the\\nevening.\\n.THU...SW wind 10 kt. Seas 8 ft. Rain in the afternoon.\\n.THU NIGHT...NE wind 10 kt. Seas 7 ft. Rain.\\n.FRI...NE wind 15 kt. Seas 7 ft.\\n.SAT...S wind 25 kt. Seas 10 ft.\\n.SUN...E wind 30 kt. Seas 12 ft.\",\n                \"instruction\": null,\n                \"response\": \"Avoid\",\n                \"parameters\": {\n                    \"AWIPSidentifier\": [\n                        \"CWFAJK\"\n                    ],\n                    \"WMOidentifier\": [\n                        \"FZAK51 PAJK 031543\"\n                    ],\n                    \"NWSheadline\": [\n                        \"SMALL CRAFT ADVISORY THROUGH LATE TONIGHT\"\n                    ],\n                    \"BLOCKCHANNEL\": [\n                        \"EAS\",\n                        \"NWEM\",\n                        \"CMAS\"\n                    ],\n                    \"VTEC\": [\n                        \"/O.NEW.PAJK.SC.Y.2860.251203T1500Z-251204T1400Z/\"\n                    ],\n                    \"eventEndingTime\": [\n                        \"2025-12-04T05:00:00-09:00\"\n                    ]\n                },\n                \"scope\": \"Public\",\n                \"code\": \"IPAWSv1.0\",\n                \"language\": \"en-US\",\n                \"web\": \"http://www.weather.gov\",\n                \"eventCode\": {\n                    \"SAME\": [\n                        \"NWS\"\n                    ],\n                    \"NationalWeatherService\": [\n                        \"SCY\"\n                    ]\n                }\n            }\n        },\n        {\n            \"id\": \"https://api.weather.gov/alerts/urn:oid:2.49.0.1.840.0.85cfcb06bd0c86092fff4359af75aac0fabec681.001.2\",\n            \"type\": \"Feature\",\n            \"geometry\": null,\n            \"properties\": {\n                \"@id\": \"https://api.weather.gov/alerts/urn:oid:2.49.0.1.840.0.85cfcb06bd0c86092fff4359af75aac0fabec681.001.2\",\n                \"@type\": \"wx:Alert\",\n                \"id\": \"urn:oid:2.49.0.1.840.0.85cfcb06bd0c86092fff4359af75aac0fabec681.001.2\",\n                \"areaDesc\": \"Waters from Pt. St. George to Cape Mendocino CA from 10 to 60 nm\",\n                \"geocode\": {\n                    \"SAME\": [\n                        \"057470\"\n                    ],\n                    \"UGC\": [\n                        \"PZZ470\"\n                    ]\n                },\n                \"affectedZones\": [\n                    \"https://api.weather.gov/zones/forecast/PZZ470\"\n                ],\n                \"references\": [],\n                \"sent\": \"2025-12-03T07:39:00-08:00\",\n                \"effective\": \"2025-12-03T07:39:00-08:00\",\n                \"onset\": \"2025-12-03T08:00:00-08:00\",\n                \"expires\": \"2025-12-03T15:45:00-08:00\",\n                \"ends\": \"2025-12-04T15:00:00-08:00\",\n                \"status\": \"Actual\",\n                \"messageType\": \"Alert\",\n                \"category\": \"Met\",\n                \"severity\": \"Minor\",\n                \"certainty\": \"Likely\",\n                \"urgency\": \"Expected\",\n                \"event\": \"Small Craft Advisory\",\n                \"sender\": \"w-nws.webmaster@noaa.gov\",\n                \"senderName\": \"NWS Eureka CA\",\n                \"headline\": \"Small Craft Advisory issued December 3 at 7:39AM PST until December 4 at 3:00PM PST by NWS Eureka CA\",\n                \"description\": \"* WHAT...North winds 15 to 25 kt with gusts up to 30 kt and seas\\n8 to 12 feet expected.\\n\\n* WHERE...Pt St George to Cape Mendocino 10 to 60 nm.\\n\\n* WHEN...Until 3 PM PST Thursday.\\n\\n* IMPACTS...Conditions will be hazardous to small craft.\",\n                \"instruction\": \"Inexperienced mariners, especially those operating smaller\\nvessels, should avoid navigating in hazardous conditions.\",\n                \"response\": \"Avoid\",\n                \"parameters\": {\n                    \"AWIPSidentifier\": [\n                        \"MWWEKA\"\n                    ],\n                    \"WMOidentifier\": [\n                        \"WHUS76 KEKA 031539\"\n                    ],\n                    \"NWSheadline\": [\n                        \"SMALL CRAFT ADVISORY IN EFFECT UNTIL 3 PM PST THURSDAY... ...GALE WARNING WILL EXPIRE AT 8 AM PST THIS MORNING\"\n                    ],\n                    \"BLOCKCHANNEL\": [\n                        \"EAS\",\n                        \"NWEM\",\n                        \"CMAS\"\n                    ],\n                    \"VTEC\": [\n                        \"/O.EXB.KEKA.SC.Y.0131.251203T1600Z-251204T2300Z/\"\n                    ],\n                    \"eventEndingTime\": [\n                        \"2025-12-04T15:00:00-08:00\"\n                    ]\n                },\n                \"scope\": \"Public\",\n                \"code\": \"IPAWSv1.0\",\n                \"language\": \"en-US\",\n                \"web\": \"http://www.weather.gov\",\n                \"eventCode\": {\n                    \"SAME\": [\n                        \"NWS\"\n                    ],\n                    \"NationalWeatherService\": [\n                        \"SCY\"\n                    ]\n                }\n            }\n        },\n        {\n            \"id\": \"https://api.weather.gov/alerts/urn:oid:2.49.0.1.840.0.85cfcb06bd0c86092fff4359af75aac0fabec681.003.1\",\n            \"type\": \"Feature\",\n            \"geometry\": null,\n            \"properties\": {\n                \"@id\": \"https://api.weather.gov/alerts/urn:oid:2.49.0.1.840.0.85cfcb06bd0c86092fff4359af75aac0fabec681.003.1\",\n                \"@type\": \"wx:Alert\",\n                \"id\": \"urn:oid:2.49.0.1.840.0.85cfcb06bd0c86092fff4359af75aac0fabec681.003.1\",\n                \"areaDesc\": \"Coastal waters from Pt. St. George to Cape Mendocino CA out 10 nm\",\n                \"geocode\": {\n                    \"SAME\": [\n                        \"057450\"\n                    ],\n                    \"UGC\": [\n                        \"PZZ450\"\n                    ]\n                },\n                \"affectedZones\": [\n                    \"https://api.weather.gov/zones/forecast/PZZ450\"\n                ],\n                \"references\": [\n                    {\n                        \"@id\": \"https://api.weather.gov/alerts/urn:oid:2.49.0.1.840.0.60f47e7d527764f0ce222d0fcb908b2519fae517.002.1\",\n                        \"identifier\": \"urn:oid:2.49.0.1.840.0.60f47e7d527764f0ce222d0fcb908b2519fae517.002.1\",\n                        \"sender\": \"w-nws.webmaster@noaa.gov\",\n                        \"sent\": \"2025-12-03T03:17:00-08:00\"\n                    }\n                ],\n                \"sent\": \"2025-12-03T07:39:00-08:00\",\n                \"effective\": \"2025-12-03T07:39:00-08:00\",\n                \"onset\": \"2025-12-03T07:39:00-08:00\",\n                \"expires\": \"2025-12-03T15:45:00-08:00\",\n                \"ends\": \"2025-12-03T22:00:00-08:00\",\n                \"status\": \"Actual\",\n                \"messageType\": \"Update\",\n                \"category\": \"Met\",\n                \"severity\": \"Minor\",\n                \"certainty\": \"Likely\",\n                \"urgency\": \"Expected\",\n                \"event\": \"Small Craft Advisory\",\n                \"sender\": \"w-nws.webmaster@noaa.gov\",\n                \"senderName\": \"NWS Eureka CA\",\n                \"headline\": \"Small Craft Advisory issued December 3 at 7:39AM PST until December 3 at 10:00PM PST by NWS Eureka CA\",\n                \"description\": \"* WHAT...North winds 5 to 15 kt with gusts up to 25 kt and seas\\n7 to 9 feet.\\n\\n* WHERE...Pt St George to Cape Mendocino out 10 nm.\\n\\n* WHEN...Until 10 PM PST this evening.\\n\\n* IMPACTS...Conditions will be hazardous to small craft.\",\n                \"instruction\": \"Inexperienced mariners, especially those operating smaller\\nvessels, should avoid navigating in hazardous conditions.\",\n                \"response\": \"Avoid\",\n                \"parameters\": {\n                    \"AWIPSidentifier\": [\n                        \"MWWEKA\"\n                    ],\n                    \"WMOidentifier\": [\n                        \"WHUS76 KEKA 031539\"\n                    ],\n                    \"NWSheadline\": [\n                        \"SMALL CRAFT ADVISORY REMAINS IN EFFECT UNTIL 10 PM PST THIS EVENING\"\n                    ],\n                    \"BLOCKCHANNEL\": [\n                        \"EAS\",\n                        \"NWEM\",\n                        \"CMAS\"\n                    ],\n                    \"VTEC\": [\n                        \"/O.CON.KEKA.SC.Y.0131.000000T0000Z-251204T0600Z/\"\n                    ],\n                    \"eventEndingTime\": [\n                        \"2025-12-03T22:00:00-08:00\"\n                    ],\n                    \"expiredReferences\": [\n                        \"w-nws.webmaster@noaa.gov,urn:oid:2.49.0.1.840.0.abe195d0561fd25b031b5bfec9df0b944a5ace40.002.1,2025-12-02T21:50:00-08:00 w-nws.webmaster@noaa.gov,urn:oid:2.49.0.1.840.0.e32ecb5cf39de3c0d1e2da73c56319d7880d5ad3.003.1,2025-12-02T15:45:00-08:00 w-nws.webmaster@noaa.gov,urn:oid:2.49.0.1.840.0.e0b91c1e8c9c801e386b75444bbd2a0bbc5299eb.003.1,2025-12-02T14:39:00-08:00 w-nws.webmaster@noaa.gov,urn:oid:2.49.0.1.840.0.0a5dc3462cdc1726ad314e876783ee5bf7071762.003.1,2025-12-02T09:55:00-08:00 w-nws.webmaster@noaa.gov,urn:oid:2.49.0.1.840.0.01de2552a96f0b556f81f7a24cea9bae9b7d39b8.003.1,2025-12-02T03:48:00-08:00 w-nws.webmaster@noaa.gov,urn:oid:2.49.0.1.840.0.ca2f9b9bc4efc4c7ec6c14c74d7b35cc28fee802.003.1,2025-12-01T20:59:00-08:00 w-nws.webmaster@noaa.gov,urn:oid:2.49.0.1.840.0.341d2d3541a24810a337eb1f7ebd4af858289c9a.003.1,2025-12-01T14:59:00-08:00\"\n                    ]\n                },\n                \"scope\": \"Public\",\n                \"code\": \"IPAWSv1.0\",\n                \"language\": \"en-US\",\n                \"web\": \"http://www.weather.gov\",\n                \"eventCode\": {\n                    \"SAME\": [\n                        \"NWS\"\n                    ],\n                    \"NationalWeatherService\": [\n                        \"SCY\"\n                    ]\n                }\n            }\n        },\n        {\n            \"id\": \"https://api.weather.gov/alerts/urn:oid:2.49.0.1.840.0.85cfcb06bd0c86092fff4359af75aac0fabec681.002.2\",\n            \"type\": \"Feature\",\n            \"geometry\": null,\n            \"properties\": {\n                \"@id\": \"https://api.weather.gov/alerts/urn:oid:2.49.0.1.840.0.85cfcb06bd0c86092fff4359af75aac0fabec681.002.2\",\n                \"@type\": \"wx:Alert\",\n                \"id\": \"urn:oid:2.49.0.1.840.0.85cfcb06bd0c86092fff4359af75aac0fabec681.002.2\",\n                \"areaDesc\": \"Waters from Cape Mendocino to Pt. Arena CA from 10 to 60 nm\",\n                \"geocode\": {\n                    \"SAME\": [\n                        \"057475\"\n                    ],\n                    \"UGC\": [\n                        \"PZZ475\"\n                    ]\n                },\n                \"affectedZones\": [\n                    \"https://api.weather.gov/zones/forecast/PZZ475\"\n                ],\n                \"references\": [],\n                \"sent\": \"2025-12-03T07:39:00-08:00\",\n                \"effective\": \"2025-12-03T07:39:00-08:00\",\n                \"onset\": \"2025-12-03T08:00:00-08:00\",\n                \"expires\": \"2025-12-03T15:45:00-08:00\",\n                \"ends\": \"2025-12-05T14:00:00-08:00\",\n                \"status\": \"Actual\",\n                \"messageType\": \"Alert\",\n                \"category\": \"Met\",\n                \"severity\": \"Minor\",\n                \"certainty\": \"Likely\",\n                \"urgency\": \"Expected\",\n                \"event\": \"Small Craft Advisory\",\n                \"sender\": \"w-nws.webmaster@noaa.gov\",\n                \"senderName\": \"NWS Eureka CA\",\n                \"headline\": \"Small Craft Advisory issued December 3 at 7:39AM PST until December 5 at 2:00PM PST by NWS Eureka CA\",\n                \"description\": \"* WHAT...North winds 15 to 25 kt with gusts up to 30 kt and seas\\n7 to 12 feet expected.\\n\\n* WHERE...Cape Mendocino to Pt Arena 10 to 60 nm.\\n\\n* WHEN...Until 2 PM PST Friday.\\n\\n* IMPACTS...Conditions will be hazardous to small craft.\",\n                \"instruction\": \"Inexperienced mariners, especially those operating smaller\\nvessels, should avoid navigating in hazardous conditions.\",\n                \"response\": \"Avoid\",\n                \"parameters\": {\n                    \"AWIPSidentifier\": [\n                        \"MWWEKA\"\n                    ],\n                    \"WMOidentifier\": [\n                        \"WHUS76 KEKA 031539\"\n                    ],\n                    \"NWSheadline\": [\n                        \"SMALL CRAFT ADVISORY IN EFFECT UNTIL 2 PM PST FRIDAY... ...GALE WARNING WILL EXPIRE AT 8 AM PST THIS MORNING\"\n                    ],\n                    \"BLOCKCHANNEL\": [\n                        \"EAS\",\n                        \"NWEM\",\n                        \"CMAS\"\n                    ],\n                    \"VTEC\": [\n                        \"/O.EXB.KEKA.SC.Y.0131.251203T1600Z-251205T2200Z/\"\n                    ],\n                    \"eventEndingTime\": [\n                        \"2025-12-05T14:00:00-08:00\"\n                    ]\n                },\n                \"scope\": \"Public\",\n                \"code\": \"IPAWSv1.0\",\n                \"language\": \"en-US\",\n                \"web\": \"http://www.weather.gov\",\n                \"eventCode\": {\n                    \"SAME\": [\n                        \"NWS\"\n                    ],\n                    
